vi "string merge with strobe.vi"(9 "Strobe String":string, 10 "Ch2 String":string, 11 "Ch1 String":string) -> (0 "Merged Output String":string, 1 "Strobe Output String":string, 2 "Ch2 Output String":string, 3 "Ch1 Output String":string)   [LabVIEW 2017]
doc: "This will calculate the needed string to send to the pulse generator for \"Channels combined\" mode, given Ch1, Ch2, and strobe strings (of possibly unlike length)."
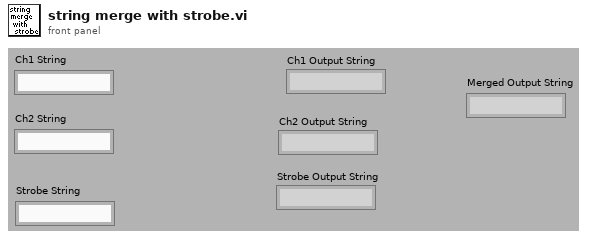
[diagram p1: front panel]
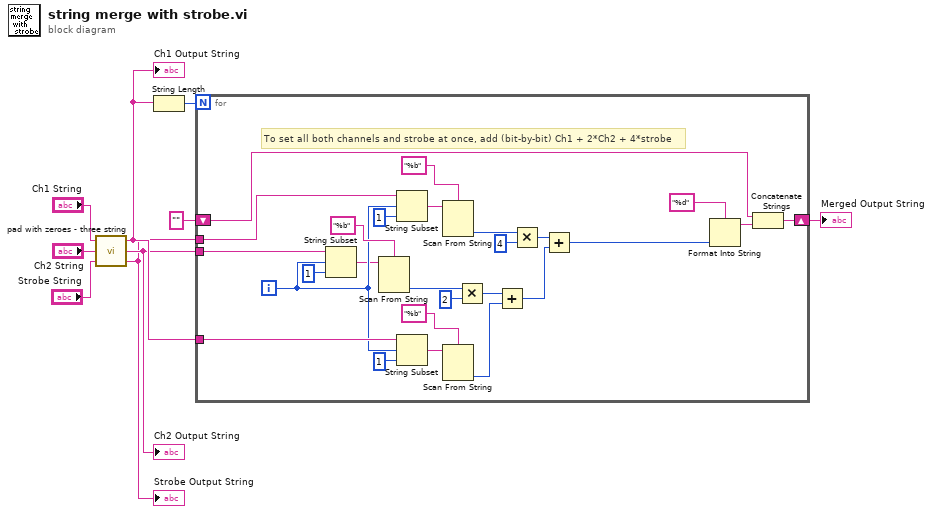
[diagram p0: block diagram]
diagram:
  n1 = call "pad with zeroes - three string.vi"("String 3 input"="Strobe String", "String 2 input"="Ch2 String", "String 1 input"="Ch1 String") -> ("String 3 output"=w1:string, "String 2 output"=w3:string, "String 1 output"=w4:string)
  "Ch1 Output String" <- w4
  "Ch2 Output String" <- w3
  "Strobe Output String" <- w1
  n2 = String Length(string=w4) -> (length=w9:i32)
  n3 = for {
    N: w9 -> [_]
    tunnel: w4 -> [w32]
    tunnel: w3 -> [w26]
    tunnel: w1 -> [w27]
    shift-right: [w13] -> w7
    shift-left: "" -> [w12]
    i -> [w25]
    # "To set all both channels and strobe at once, add (bit-by-bit) Ch1 + 2*Ch2 + 4*strobe"
    n4 = String Subset(string=w26, offset (0)=w25, length (rest)=1 ("length (rest)")) -> (substring=w23:string)
    n5 = Scan From String(format string="%b", input string=w23) -> (output 1=w20:i32)  [unwired: 2 in, 4 out]
    n6 = String Subset(string=w27, offset (0)=w25, length (rest)=1 ("length (rest)")) -> (substring=w24:string)
    n7 = String Subset(string=w32, offset (0)=w25, length (rest)=1 ("length (rest)")) -> (substring=w30:string)
    n8 = Scan From String(format string="%b", input string=w24) -> (output 1=w11:i32)  [unwired: 2 in, 4 out]
    n9 = Scan From String(format string="%b", input string=w30) -> (output 1=w10:i32)  [unwired: 2 in, 4 out]
    n10 = Multiply(x=w20, y=i8 2) -> (x*y=w19:i32)
    n11 = Add(x=w19, y=w10) -> (x+y=w18:i32)
    n12 = Multiply(x=w11, y=i8 4) -> (x*y=w17:i32)
    n13 = Add(x=w17, y=w18) -> (x+y=w15:i32)
    n14 = Format Into String(format string="%d", w15) -> (resulting string=w14:string)  [unwired: 2 in, 1 out]
    n15 = Concatenate Strings(w12, w14) -> (w13:string)
  }
  "Merged Output String" <- w7
